vi "SaveAsync.vi"(8 "error in (no error)":errorcluster, 10 "Path":path, 11 "Source":T1) -> (0 "error out":errorcluster)   [LabVIEW 2019, in "VisionUI.lvlib" / "VisionUI.lvclass"]
uses:
  VisionUI.lvclass
  <vilib>/vision/Image Controls.llb/IMAQ Image.ctl
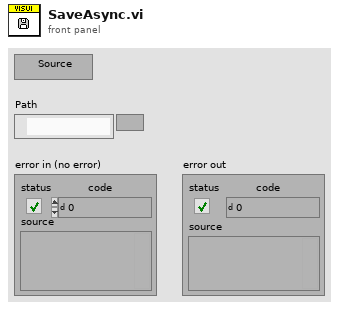
[diagram p1: front panel]
types:
  T1 = typedef "IMAQ Image.ctl" = refnum<image>
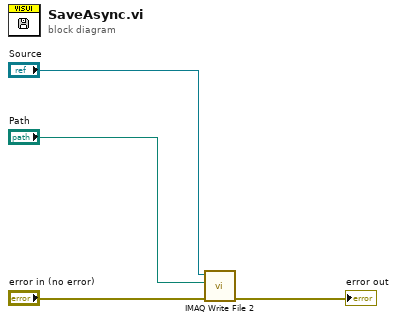
[diagram p0: block diagram]
diagram:
  n1 = call-poly "IMAQ Write File 2"("error in (no error)"="error in (no error)", "File Path"="Path", "Image"="Source") -> ("error out"=→"error out":errorcluster)  [unwired: 7 in, 1 out]
